vi "XY_Built_History.vi"(0 "input x":dbl[](array[numeric])=[0.0, 0.0, 0.0], 1 "input y":dbl[](array[numeric])=[0.0, 0.0, 0.0]) -> (6 "xo":sgl[][](array[numeric]), 7 "yo":sgl[][](array[numeric]))   [LabVIEW 2011]
uses:
  <vilib>/imath/engines/lvmath2/RunTimeEngine/ErrorHandling/NIMS_Finalize Error.vi
  <vilib>/imath/engines/lvmath2/RunTimeEngine/RangeToken/NIMS_Range_R2.vi
  <vilib>/imath/engines/lvmath2/RunTimeEngine/VariableToken/Read/NIMS_Get Elements - SorM(_,$) - Check.vi
  <instcachedir>/0/NIMS_Get Elements - SorM(_,$) - Check_3B494CC2A76E49EA8E6F8F732E2632C3.lvgen/NIMS_Get Elements - SorM(_,$) - Check_3B494CC2A76E49EA8E6F8F732E2632C3_001.vi
  <vilib>/imath/engines/lvmath2/RunTimeEngine/MatrixToken/NIMS_MatrixToken_M_RV.vi
  <instcachedir>/0/NIMS_MatrixToken_M_RV_E824F4BEDD6A482A8DA68759FEA3999F.lvgen/NIMS_MatrixToken_M_RV_E824F4BEDD6A482A8DA68759FEA3999F_001.vi
  <vilib>/imath/engines/lvmath2/RunTimeEngine/ErrorHandling/NIMS_Create Error From Enums.vi
  <vilib>/imath/engines/lvmath2/RunTimeEngine/NodeEndStatement/NIMS_NodeEndStatement_Output.vi
  <instcachedir>/0/NIMS_NodeEndStatement_Output_53EC0D466D134D7ABD903AC30B43404B.lvgen/NIMS_NodeEndStatement_Output_53EC0D466D134D7ABD903AC30B43404B_002.vi
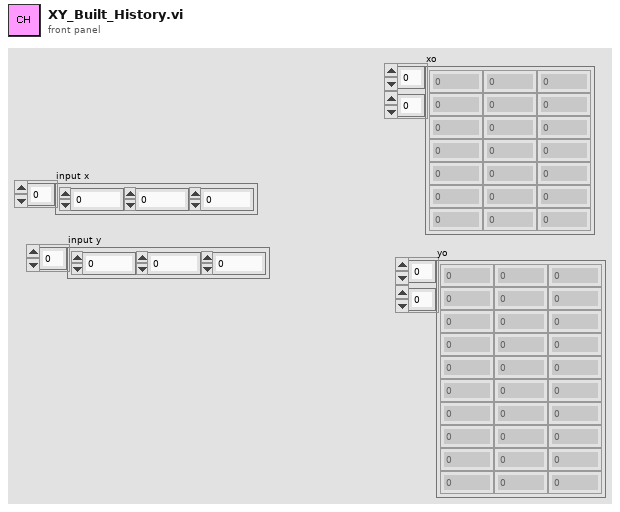
[diagram p1: front panel]
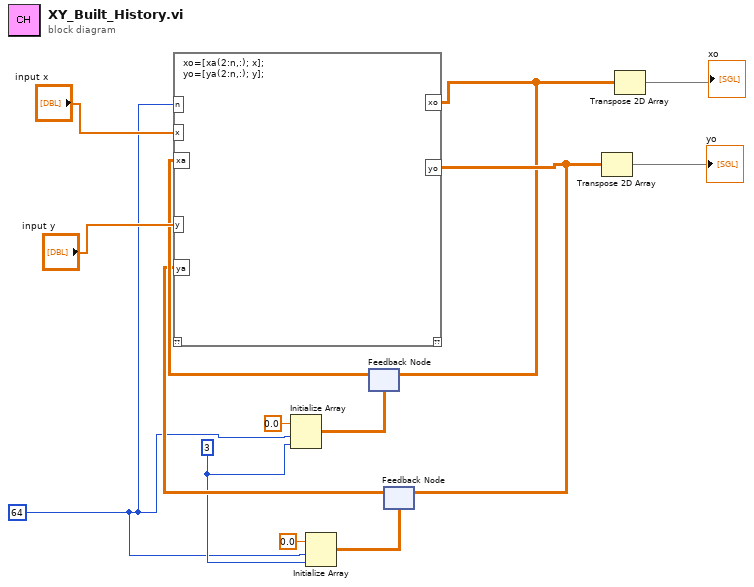
[diagram p0: block diagram]
diagram:
  w5 = 3 ("dimension size")
  w4 = 64 ("dimension size")
  n1 = Initialize Array(sgl 0.0 ("element"), w4, w5) -> (w11:sgl[][])
  n2 = Initialize Array(sgl 0.0 ("element"), w4, w5) -> (w9:sgl[][])
  n3 = feedback #1(w11) -> (w8:dbl[][])
  n4 = feedback #2(w9) -> (w7:dbl[][])
  n5 = mathscript code="xo=[xa(2:n,:); x];\nyo=[ya(2:n,:); y];"("x"="input x", "y"="input y", "xa"=w8, "ya"=w7, "n"=w4) -> ("yo"=w6:dbl[][], "xo"=w3:dbl[][])  [unwired: 1 in, 1 out]
  n6 = feedback-in #1(w3) -> ()
  n7 = feedback-in #2(w6) -> ()
  n8 = Transpose 2D Array(2D array=w6) -> (transposed array=→"yo":dbl[][])
  n9 = Transpose 2D Array(2D array=w3) -> (transposed array=→"xo":dbl[][])
